vi "UpdateBroadcastCounter.vi"(9 "BroadcastCounter":u8, 10 "Code67Memory":refnum<k21>, 11 "Code66Memory":refnum<k21>) -> ()   [LabVIEW 2016, in "FPGAMockMDILC.lvlib"]
uses:
  FPGAMockMDILC.lvlib
  <vilib>/rvi/Emulation/niFpgaSctlEmulationGetInTimedLoop.vi
  <vilib>/Utility/error.llb/Clear Errors.vi
  <vilib>/rvi/DataTransferAndStorage/Container/Common/niFpgaContainerExecOnDevCompGetState.vi
  <vilib>/rvi/Emulation/niFpgaEmulationIsFPGAContextNoSignature.vi
  <vilib>/rvi/DataTransferAndStorage/Container/Common/niFpgaContainerGetUniqueNameForEmu.vi
  <vilib>/rvi/Emulation/niFpgaProcessEmulError.vi
  <vilib>/rvi/errors/nirviReportUnexpectedCaseInternalError (U32).vi
  <vilib>/rvi/Memory/Memory_Emulation/niFpgaMemoryEmulationCacheClearOnFirstRun.vi
  <vilib>/rvi/Memory/Memory_Emulation/nirvimemoryEmulationManagerCache_MakeExclusive.vi
  <vilib>/rvi/Memory/Memory_Emulation/niFpgaMemoryEmulationValidateCache.vi
  <vilib>/rvi/Memory/Memory_Emulation/nirvimemoryEmulationManagerCache_InsertValue.vi
  <vilib>/rvi/Memory/Memory_Emulation/nirvimemoryEmulationManagerCache_ReleaseExclusive.vi
  <vilib>/rvi/Memory/Memory_Emulation/nirvimemoryEmulationManagerCache_GetValue.vi
  <vilib>/rvi/Memory/Memory_Emulation/nirvimemoryEmulationManagerCache_SetValue.vi
  <vilib>/rvi/Emulation/niFpgaSctlEmulationResourceMgr.vi
  <vilib>/rvi/DataTransferAndStorage/Container/XNode/niFpgaContainer.xnode
  <vilib>/rvi/Memory/Memory_Emulation/niFpgaMemoryEmulationRefIn.vi
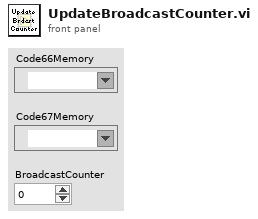
[diagram p1: front panel]
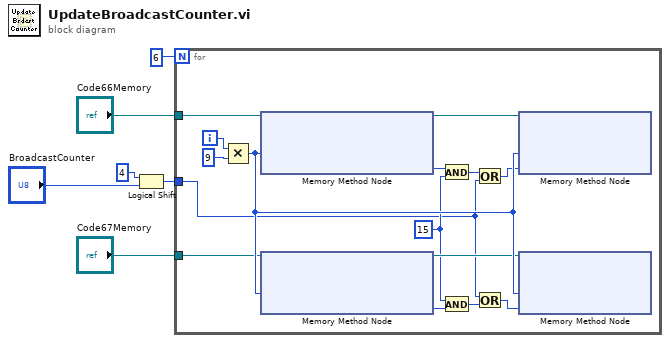
[diagram p0: block diagram]
diagram:
  n1 = Logical Shift(y=i16 4, x="BroadcastCounter") -> (x << y=w1:u8)
  n2 = for {
    N: 6 -> [_]
    tunnel: w1 -> [w7]
    tunnel: "Code66Memory" -> [w16]
    tunnel: "Code67Memory" -> [w15]
    i -> [w21]
    w12 = u8 15 ("y")
    n3 = Multiply(x=w21, y=9) -> (x*y=w19:i32)
    n4 = xnode ("Memory Method Node")("Address"=w19, "Memory In"=w16) -> ("Data"=w14:u8, "Memory Out"=w18:refnum<k21>)
    n5 = xnode ("Memory Method Node")("Address"=w19, "Memory In"=w15) -> ("Data"=w13:u8, "Memory Out"=w17:refnum<k21>)
    n6 = And(x=w14, y=w12) -> (x .and. y?=w11:u8)
    n7 = And(x=w12, y=w13) -> (x .and. y?=w9:u8)
    n8 = Or(x=w11, y=w7) -> (x .or. y?=w10:u8)
    n9 = Or(x=w7, y=w9) -> (x .or. y?=w8:u8)
    n10 = xnode ("Memory Method Node")("Address"=w19, "Data"=w10, "Memory In"=w18) -> ()  [unwired: 1 out]
    n11 = xnode ("Memory Method Node")("Address"=w19, "Data"=w8, "Memory In"=w17) -> ()  [unwired: 1 out]
  }
